vi "1ST VI.vi"() -> ()   [LabVIEW 2018]
panel:
  out "Numeric Indicator":dbl
  out "Y=((A^2+B^2)(1+E)+CD)":dbl
  in  "E":dbl
  in  "D":i32
  in  "C":dbl
  in  "B":dbl
  in  "A":dbl
  # "Evaluting Boolean Expresions"
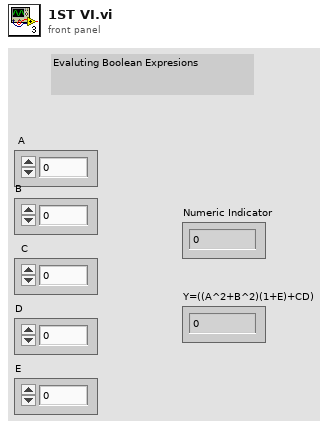
[diagram p1: front panel]
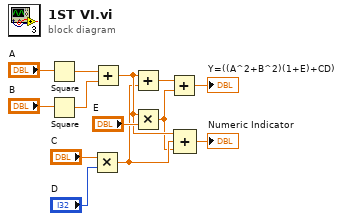
[diagram p0: block diagram]
diagram:
  n1 = Square(x="A") -> (x^2=w13:dbl)
  n2 = Square(x="B") -> (x^2=w12:dbl)
  n3 = Multiply(x="C", y="D") -> (x*y=w3:dbl)
  n4 = Add(x=w13, y=w12) -> (x+y=w4:dbl)
  n5 = Add(x=w4, y=w3) -> (x+y=w11:dbl)
  n6 = Multiply(x=w4, y="E") -> (x*y=w2:dbl)
  n7 = Add(x=w11, y=w2) -> (x+y=→"Y=((A^2+B^2)(1+E)+CD)":dbl)
  n8 = Compound Arithmetic op=ADD(w4, w3, w2) -> (→"Numeric Indicator":dbl)
